vi "LocationFromCamera.vi"(8 "error in":errorcluster, 11 "Image Path":T2) -> (0 "error out":errorcluster, 1 "Valid?":bool, 2 "Angle":sgl, 3 "Location":T1 {"North" format="%#_10f"; "East" format="%#_8f"})   [LabVIEW 2013]
doc: "This VI will find the tug with the symbol for the greek letter which is passed. It accepts the pool image and the templete image for the greek letter passed. It outputs the the X and Y location in camera pixels and the heading in degrees. The valid? line indicates the tug was found. If the data is not valid it outputs -1's."
uses:
  <vilib>/vision/Image Controls.llb/IMAQ Image.ctl
  Data/TypeDefs/UTM Location.ctl
panel:
  out "Matches":T3(array[cluster]) {"Bounding Box"."y" format="%.2f"; "Bounding Box"."x" format="%.2f"; "Position"."y" format="%.2f"; "Position"."x" format="%.2f"; "Score" format="%.2f"; "Scale" format="%.2f"; "Angle" format="%.2f"}
  out "Template Image":T2(plugin-control)
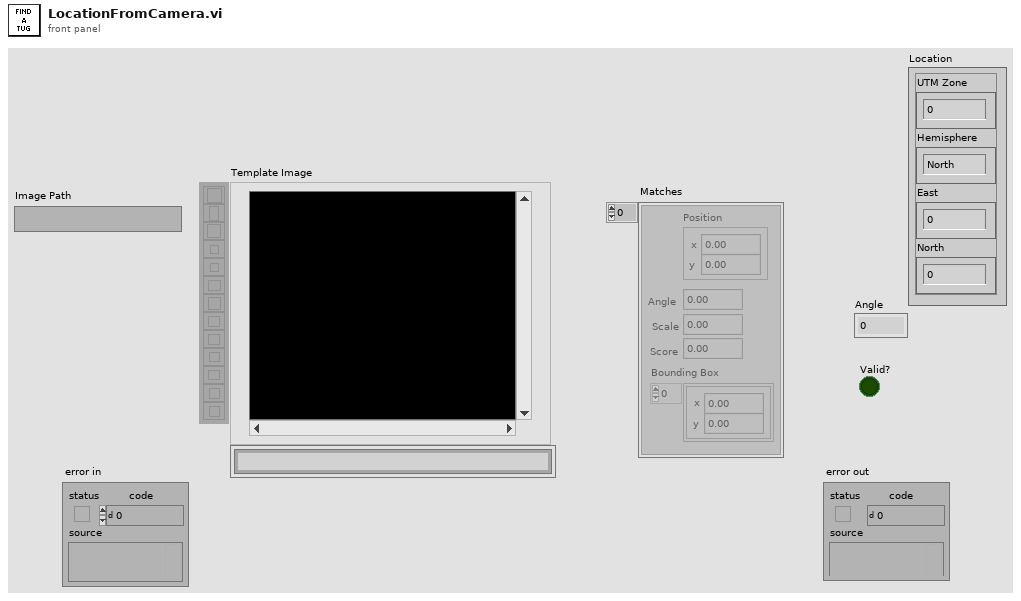
[diagram p1: front panel]
types:
  T1 = typedef "UTM Location.ctl" = cluster{"UTM Zone":dbl, "Hemisphere":enum16{"North", "South"}, "East":dbl, "North":dbl}
  T2 = typedef "IMAQ Image.ctl" = refnum<image>
  T3 = cluster{"Position":cluster{"x":sgl, "y":sgl}, "Angle":sgl, "Scale":sgl, "Score":sgl, "Bounding Box":cluster{"x":sgl, "y":sgl}[]}[]
  T4 = cluster{"Global Rectangle":i32[], "Contours":cluster{"ID":enum32{"External", "Internal"}, "Type":u32, "Coordinates":i32[]}[]}
  T5 = typedef "Image Type" = u32
  T6 = cluster{"Match Mode (Pattern Matching 1)":u16, "Subpixel Accuracy (Pattern Matching 1)":bool, "Rotation Angle Ranges (degrees) (Pattern Matching 1)":cluster{sgl, sgl}[]}
  T7 = cluster{"ROI Descriptor (Pattern Matching 1)":cluster{"Global Rectangle":i32[], "Contours":cluster{"ID":enum32{"External", "Internal"}, "Type":u32, "Coordinates":i32[]}[]}, "Number of Matches Requested (Pattern Matching 1)":i32, "Minimum Match Score (Pattern Matching 1)":sgl}
  T8 = cluster{"Position":cluster{"x":sgl, "y":sgl}, "Angle":sgl, "Scale":sgl, "Score":sgl, "Bounding Box":cluster{"x":sgl, "y":sgl}[]}
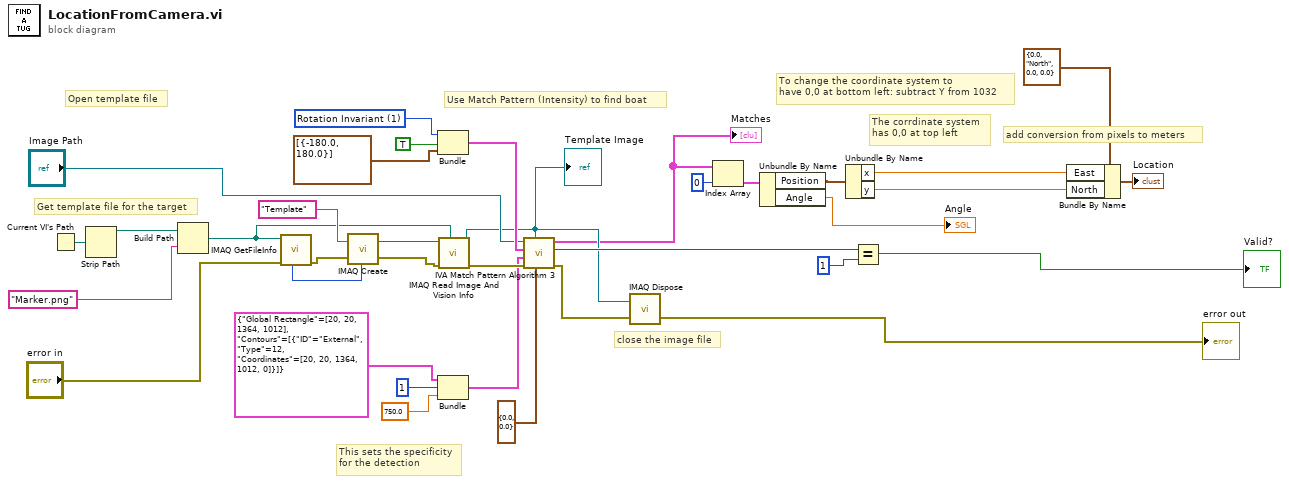
[diagram p0: block diagram]
diagram:
  w36 = u16 1 items=["Shift Invariant", "Rotation Invariant"] ("Match Mode (Pattern Matching 1)")
  # "add conversion from pixels to meters"
  # "This sets the specificity\nfor the detection"
  # "To change the coordinate system to \nhave 0,0 at bottom left: subtract Y from 1032"
  # "The corrdinate system\nhas 0,0 at top left"
  # "close the image file"
  # "Use Match Pattern (Intensity) to find boat"
  # "Open template file"
  # "Get template file for the target"
  n1 = Current VI's Path() -> (path=w30:path)
  n2 = Strip Path(path=w30) -> (stripped path=w29:path)  [unwired: 1 out]
  n3 = Build Path(base path=w29, name or relative path="Marker.png") -> (appended path=w25:path)
  n4 = call "IMAQ GetFileInfo"("error in (no error)"="error in", "File Path"=w25) -> ("error out"=w28:errorcluster, "Image Type"=w27:T5)  [unwired: 3 in, 5 out]
  n5 = call "IMAQ Create"("Image Name"="Template", "Image Type"=w27, "error in (no error)"=w28) -> ("New Image"=w23:T2, "error out"=w24:errorcluster)  [unwired: 1 in, 1 out]
  n6 = Bundle("Match Mode (Pattern Matching 1)"=w36, "Subpixel Accuracy (Pattern Matching 1)"=TRUE, "Rotation Angle Ranges (degrees) (Pattern Matching 1)"=cluster{sgl, sgl}[] [{-180.0, 180.0}]) -> (w20:T6)  [unwired: 1 out]
  n7 = Bundle("ROI Descriptor (Pattern Matching 1)"=T4 {"Global Rectangle"=[20, 20, 1364, 1012], "Contours"=[{"ID"=enum."External", "Type"=12, "Coordinates"=[20, 20, 1364, 1012, 0]}]}, "Number of Matches Requested (Pattern Matching 1)"=1, "Minimum Match Score (Pattern Matching 1)"=sgl 750.0) -> (w21:T7)  [unwired: 1 out]
  n8 = call "IMAQ Read Image And Vision Info"("File Path"=w25, "error in (no error)"=w24, "Image"=w23) -> ("error out"=w22:errorcluster, "Image Out"=w8:T2)  [unwired: 1 in, 6 out]
  "Template Image" <- w8
  n9 = call <vilib>:"IVA Match Pattern Algorithm 3.vi"("Match Offset"=cluster{"X":sgl, "Y":sgl} {"X"=0.0, "Y"=0.0} ("Match Offset (Pattern Matching 1)"), "Image Template"=w8, "error in (no error)"=w22, "Match Parameters"=w21, "Setup Match Parameters"=w20, "Image"="Image Path") -> ("error out"=w12:errorcluster, "Number of Matches"=w16:i32, "Matches"=w7:T3)  [unwired: 3 out]
  "Matches" <- w7
  n10 = call "IMAQ Dispose"("Image"=w8, "error in (no error)"=w12) -> ("error out"=→"error out":errorcluster)  [unwired: 4 in]
  n11 = Index Array(array=w7, index=0) -> (element=w18:T8)
  n12 = Unbundle By Name(w18) -> ("Position"=w17:cluster{"x":sgl, "y":sgl}, "Angle"=→"Angle":sgl)
  n13 = Unbundle By Name(w17) -> ("x"=w3:sgl, "y"=w2:sgl)
  n14 = Equal?(x=w16, y=1) -> (x = y?=→"Valid?":bool)
  n15 = Bundle By Name(cluster=T1 {"UTM Zone"=0.0, "Hemisphere"=enum."North", "East"=0.0, "North"=0.0} ("UTM Location"), "East"=w3, "North"=w2) -> (→"Location":T1)
